vi "ConnectUDP.vi"(11 "FPGA in":refnum<queue>) -> (2 "Connected":bool, 3 "FPGA out":refnum<queue>)   [LabVIEW 2019, in "FPGA.lvlib"]
uses:
  FPGA.lvlib
  FPGA.ctl
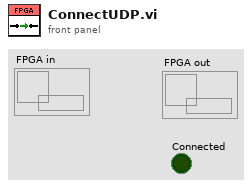
[diagram p1: front panel]
types:
  T1 = typedef "FPGA.lvlib/FPGA.ctl" = cluster{"Start freq. [Hz]":dbl, "Sweep duration [s]":dbl, "Freq. step [Hz]":dbl, "DAC Sample Rate":dbl, "ADC Sample Rate":dbl, "CMD port":u16, "DFAST port":u16, "CMD ID":refnum<k16>, "DFAST ID":refnum<k16>, "CMD error out":errorcluster, "FPGA IP":string, "DFAST error out ":errorcluster, "Stop freq. [Hz]":dbl, "Discrete sweep":bool, "Initial NCO":u32, "Difference NCO":i32, "step NCO":i64, "Final NCO":u32, "clocks for step":u32, "demodulation":bool, "NCO Phase Precision":u32, "NCO Sample Rate":dbl, "Time for step [s]":dbl, "NCO freq. resolution":dbl, "Sweep speed [Hz/s]":dbl, "Connected":bool, "Slew Rate [V/us]":dbl, "Parameters_ok":bool, "Amplitude [mVpp]":dbl, "Scale Factor":fxp<+,16,0>, "Acquiring":bool, "DAC-ADC Latency":u16, "Digital Gain":i32, "Number of steps":i32, "Averaging preferred":bool, "Filter Order":u32, "Settling":enum16{"99%", "99,9%"}}
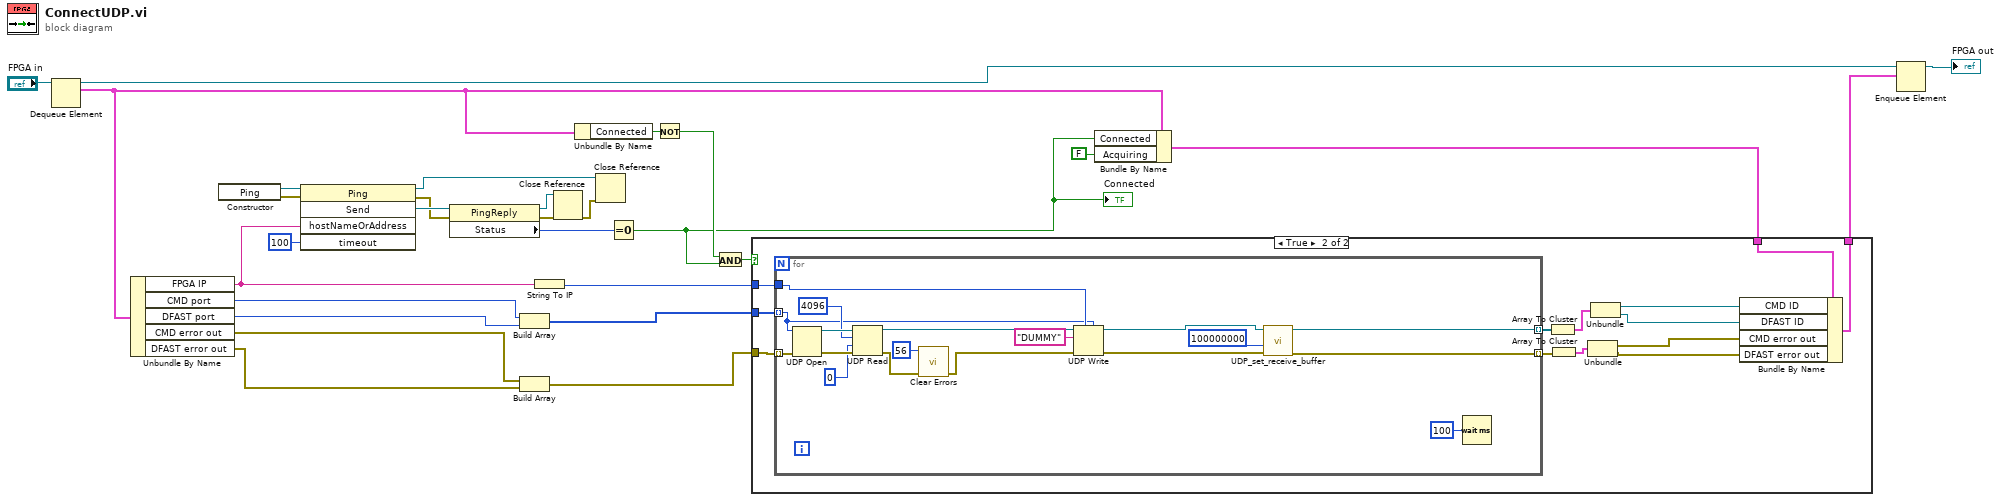
[diagram p0: block diagram]
diagram:
  n1 = Dequeue Element(queue="FPGA in") -> (queue out=w9:refnum<queue>, element=w5:T1)  [unwired: 2 in, 2 out]
  n2 = Unbundle By Name(w5) -> ("FPGA IP"=w14:string, "CMD port"=w29:u16, "DFAST port"=w28:u16, "CMD error out"=w26:errorcluster, "DFAST error out"=w25:errorcluster)
  n3 = constructor class="Ping"() -> (reference out=w15:refnum<k24>, error out=w16:errorcluster)  [unwired: 3 in, 1 out]
  n4 = invoke class="Ping" method="Send"(reference=w15, error in=w16, "hostNameOrAddress"=w14, "timeout"=100) -> (reference out=w23:refnum<k24>, error out=w17:errorcluster, "Send"=w18:refnum<k24>)  [unwired: 1 in, 2 out]
  n5 = property class="PingReply"(reference=w18, error in=w17) -> (reference out=w21:refnum<k24>, error out=w20:errorcluster, "Status"=w19:i32)
  n6 = Build Array(w29, w28) -> (w7:u16[])
  n7 = Build Array(w26, w25) -> (w24:errorcluster[])
  n8 = String To IP(1:w14) -> (0:w27:u32)
  n9 = Close Reference(reference=w21, error in (no error)=w20) -> (error out=w22:errorcluster)
  n10 = Unbundle By Name(w5) -> ("Connected"=w4:bool)
  n11 = Close Reference(reference=w23, error in (no error)=w22) -> ()  [unwired: 1 out]
  n12 = Equal To 0?(x=w19) -> (x = 0?=w2:bool)
  "Connected" <- w2
  n13 = Not(x=w4) -> (.not. x?=w3:bool)
  n14 = And(x=w3, y=w2) -> (x .and. y?=w1:bool)
  n15 = Bundle By Name(cluster=w5, "Connected"=w2, "Acquiring"=FALSE) -> (w8:T1)
  n16 = case shown="True" w1 {
    tunnel: w8 -> [w30 w39]
    tunnel: [w30 w40] -> w10
    tunnel: w24 -> [_ w42]
    tunnel: w27 -> [_ w43]
    tunnel: w7 -> [_ w41]
    frame False {
    }
    frame True {
      n17 = for {
        tunnel: [w61] -> w38 mode=indexing
        tunnel: w43 -> [w58]
        tunnel: [w60] -> w37 mode=indexing
        tunnel: w42 -> [w59] mode=indexing
        tunnel: w41 -> [w45] mode=indexing
        n18 = UDP Open(8:w59, 11:w45) -> (port=w55:refnum<k16>, 0:w56:errorcluster)  [unwired: 3 in, 1 out]
        n19 = UDP Read(connection ID=w55, max size (548)=4096, timeout ms (25000)=0, 8:w56) -> (error out=w52:errorcluster, 3:w57:refnum<k16>)  [unwired: 3 out]
        n20 = call <vilib>:"Clear Errors.vi"("error in (no error)"=w52, "specific error code to clear (0: all)"=56) -> ("error out"=w50:errorcluster)  [unwired: 4 in, 1 out]
        n21 = UDP Write(address=w58, port or service name=w45, connection ID=w57, data in="DUMMY", 8:w50) -> (error out=w46:errorcluster, 3:w47:refnum<k16>)  [unwired: 1 in]
        n22 = call "UDP_set_receive_buffer.vi"("error in (no error)"=w46, "Receive Buffer Size"=u32 100000000, "connection ID"=w47) -> ("error out"=w60:errorcluster, "connection ID out"=w61:refnum<k16>)  [unwired: 6 in]
        n23 = Wait (ms)(milliseconds to wait=u32 100) -> ()  [unwired: 1 out]
      }
      n24 = Array To Cluster(array=w38) -> (cluster=w36:cluster{"[0]":refnum<k16>, "[1]":refnum<k16>})
      n25 = Array To Cluster(array=w37) -> (cluster=w35:cluster{"[0]":errorcluster, "[1]":errorcluster})
      n26 = Unbundle(w35) -> ("[0]"=w34:errorcluster, "[1]"=w33:errorcluster)
      n27 = Unbundle(w36) -> ("[0]"=w32:refnum<k16>, "[1]"=w31:refnum<k16>)
      n28 = Bundle By Name(cluster=w39, "CMD ID"=w32, "DFAST ID"=w31, "CMD error out"=w34, "DFAST error out"=w33) -> (w40:T1)
    }
  }
  n29 = Enqueue Element(queue=w9, element=w10) -> (queue out=→"FPGA out":refnum<queue>)  [unwired: 2 in, 2 out]
